vi "convertTimingCluster.vi"(8 "error in (no error)":errorcluster, 10 "Timing":T5, 11 "DIO64Output in":refnum<class "DIO64Output.lvclass">) -> (0 "error out":errorcluster, 2 "Out Config Control":T1 {"#transitions" format="%.0x"; "repetitions" format="%.0x"; "DAQ clock modulo" format="%.0x"}, 3 "DIO64Output out":refnum<class "DIO64Output.lvclass">)   [LabVIEW 2009, in "Hardware.lvlib" / "Channels.lvlib" / "DIO64Output.lvclass"]
uses:
  DIO64Output.lvclass
  <userlib>/dio64_32.LLB/DIO64 Out Config Control.ctl
  <userlib>/dio64_32.LLB/DIO64 clock control.ctl
  <userlib>/dio64_32.LLB/DIO64 start trig.ctl
  <userlib>/dio64_32.LLB/DIO64 stop trig.ctl
panel:
  in  "Out Config dumpy":T1 {"#transitions" format="%.0x"; "repetitions" format="%.0x"; "DAQ clock modulo" format="%.0x"}
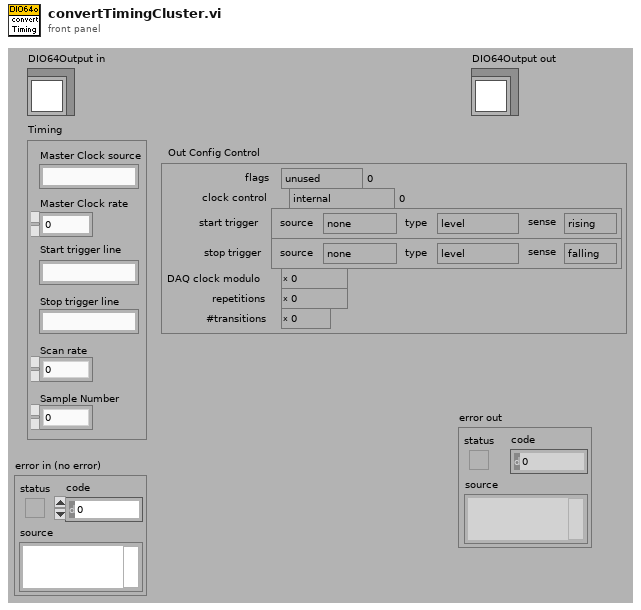
[diagram p1: front panel]
types:
  T1 = typedef "DIO64 Out Config Control.ctl" = cluster{"flags":enum16{"unused"}, "clock control":T2, "start trigger":T3, "stop trigger":T4, "DAQ clock modulo":u32, "repetitions":u32, "#transitions":u16}
  T2 = typedef "DIO64 clock control.ctl" = enum16{"internal", "external", "trig 0", "OCXO"}
  T3 = typedef "DIO64 start trig.ctl" = cluster{"source":enum16{"none", "internal", "external", "trig 2", "PXI Star"}, "type":enum16{"level", "edge", "edge to edge"}, "sense":enum16{"rising", "falling"}}
  T4 = typedef "DIO64 stop trig.ctl" = cluster{"source":enum16{"none", "internal", "external", "trig 3 in", "output FIFO"}, "type":enum16{"level", "edge"}, "sense":enum16{"falling", "rising"}}
  T5 = cluster{"Master Clock source":string, "Master Clock rate":dbl, "Start trigger line":string, "Scan rate":dbl, "Stop trigger line":string, "Sample Number":dbl}
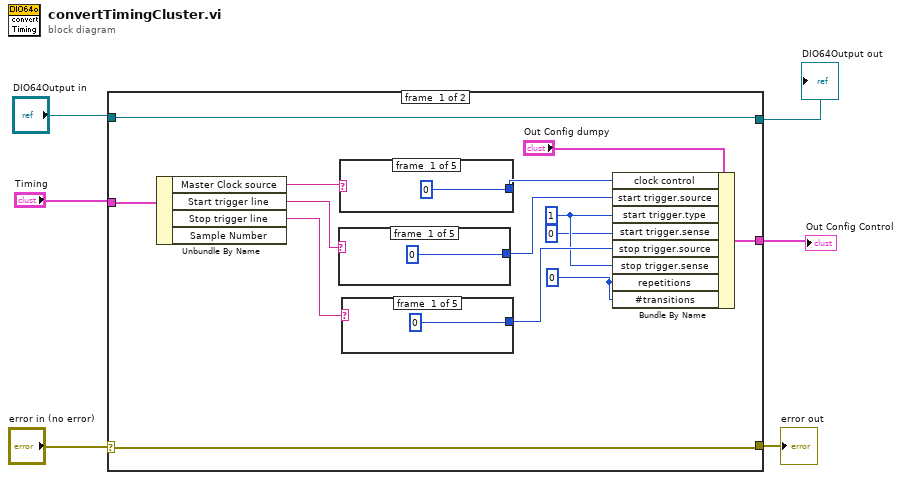
[diagram p0: block diagram]
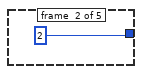
[diagram p2: hidden frame]
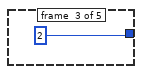
[diagram p3: hidden frame]
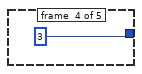
[diagram p4: hidden frame]
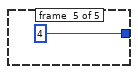
[diagram p5: hidden frame]
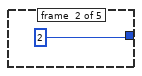
[diagram p6: hidden frame]
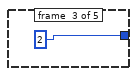
[diagram p7: hidden frame]
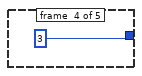
[diagram p8: hidden frame]
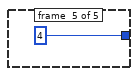
[diagram p9: hidden frame]
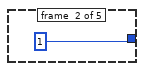
[diagram p10: hidden frame]
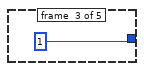
[diagram p11: hidden frame]
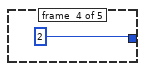
[diagram p12: hidden frame]
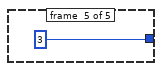
[diagram p13: hidden frame]
diagram:
  n1 = case shown="No Error" "error in (no error)" {
    selector: "error in (no error)" -> [w8 w37]
    tunnel: [w8 w37] -> w5
    tunnel: [w9 w36] -> w3
    tunnel: "DIO64Output in" -> [w9 w36]
    tunnel: "Timing" -> [w20 _]
    tunnel: [w10 _] -> w1
    frame #0 {
      w7 = 0
      w12 = 1
      n2 = Unbundle By Name(w20) -> ("Master Clock source"=w19:string, "Start trigger line"=w16:string, "Stop trigger line"=w14:string)  [unwired: 1 out]
      n3 = case shown="\"external\"" w16 {
        tunnel: [0 2 2 3 4] -> w15
        frame #0 {
        }
        frame #1 {
        }
        frame #2 {
        }
        frame #3 {
        }
        frame #4 {
        }
      }
      n4 = case shown="\"PXI_Trig_00\"" w19 {
        tunnel: [0 1 1 2 3] -> w17
        frame #0 {
        }
        frame #1 {
        }
        frame #2 {
        }
        frame #3 {
        }
        frame #4 {
        }
      }
      n5 = case shown="\"none\", Default" w14 {
        tunnel: [0 2 2 3 4] -> w13
        frame #0 {
        }
        frame #1 {
        }
        frame #2 {
        }
        frame #3 {
        }
        frame #4 {
        }
      }
      n6 = Bundle By Name(cluster="Out Config dumpy", "clock control"=w17, "start trigger.source"=w15, "start trigger.type"=w12, "start trigger.sense"=0, "stop trigger.source"=w13, "stop trigger.sense"=w12, "repetitions"=w7, "#transitions"=w7) -> (w10:T1)
    }
    frame #1 {
    }
  }
  "error out" <- w5
  "DIO64Output out" <- w3
  "Out Config Control" <- w1
